vi "CLD 10 CSV file utility_exercise.vi"(8 "Error In":errorcluster, 10 "CLD 10 file Enum":T2, 11 "[Data In]":T1[](array[typedef])=[{"Step Time Target"=3, "Step 1"=TRUE, "Step 2"=FALSE, "Step 3"=FALSE}, {"Step Time Target"=4, "Step 1"=FALSE, "Step 2"=TRUE, "Step 3"=FALSE}, {"Step Time Target"=5, "Step 1"=FALSE, "Step 2"=FALSE, "Step 3"=TRUE}]) -> (0 "Error Out":errorcluster, 3 "[Data Out]":T1[](array[typedef]))   [LabVIEW 2025]
uses:
  CLD 10 CSV file data structure.ctl
  CLD 10 CSV file enum.ctl
  <vilib>/Utility/file.llb/Read Delimited Spreadsheet (string).vi
  <vilib>/Utility/file.llb/Write Delimited Spreadsheet (string).vi
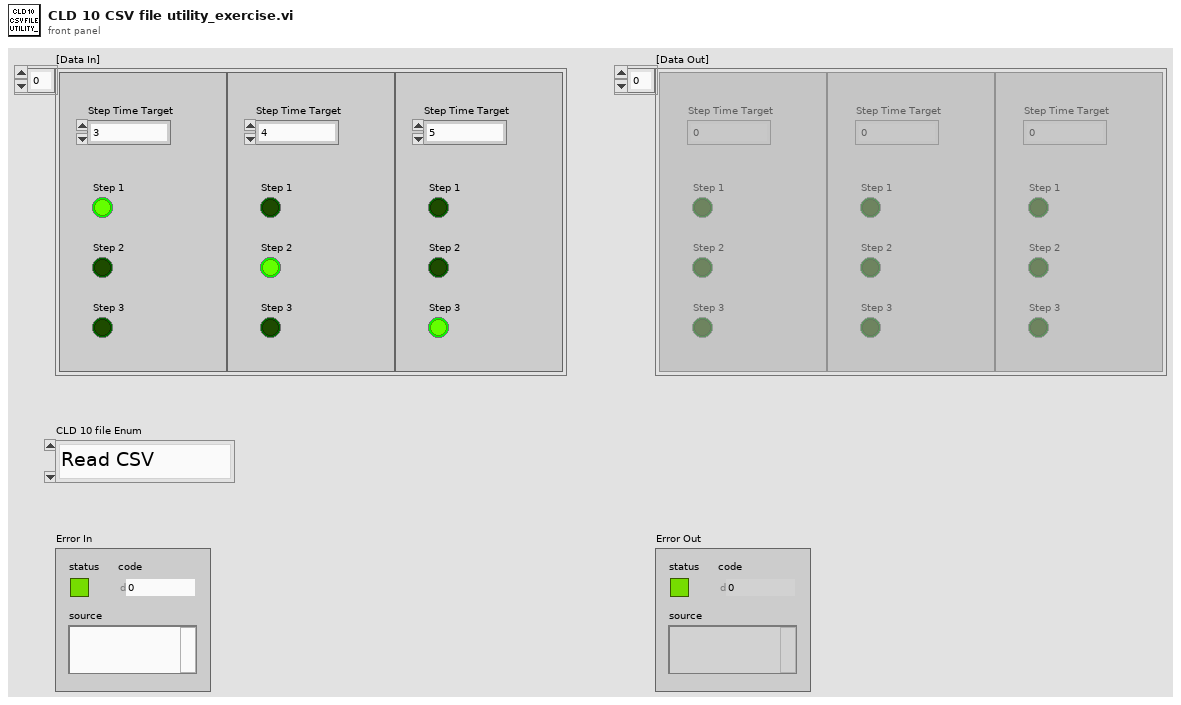
[diagram p1: front panel]
types:
  T1 = typedef "CLD 10 CSV file data structure.ctl" = cluster{"Step Time Target":i32, "Step 1":bool, "Step 2":bool, "Step 3":bool}
  T2 = typedef "CLD 10 CSV file enum.ctl" = enum16{"Read CSV", "Write CSV"}
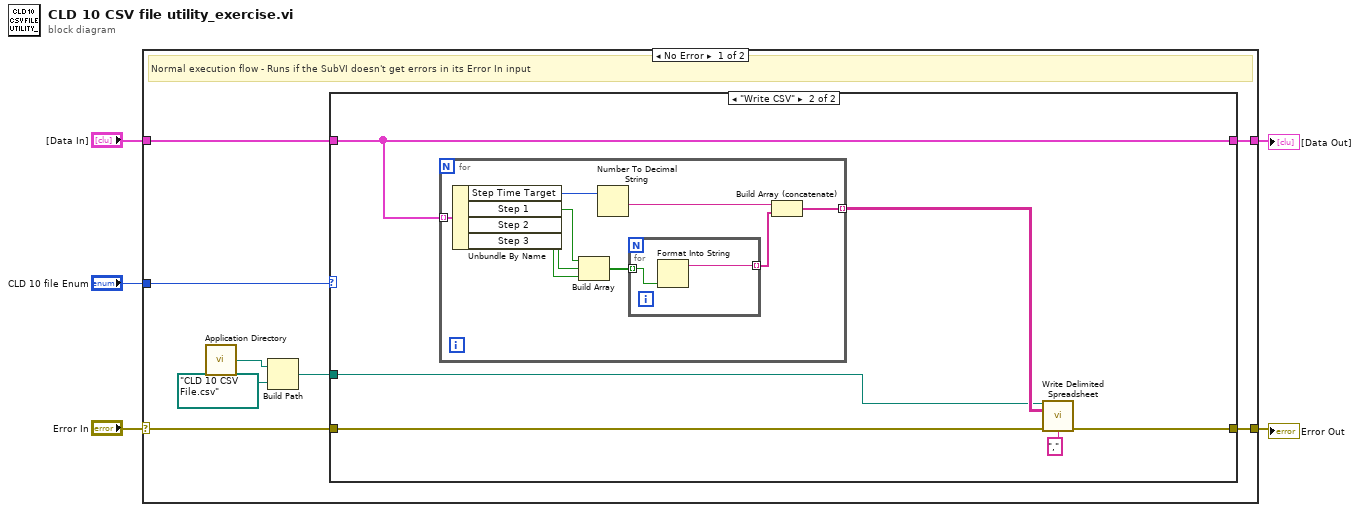
[diagram p0: block diagram]
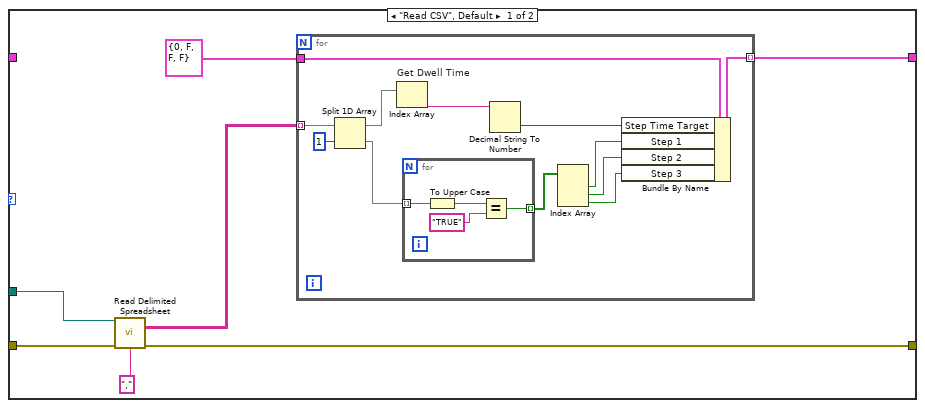
[diagram p2: hidden frame]
diagram:
  n1 = case shown="No Error" "Error In" {
    selector: "Error In" -> [w13 w55]
    tunnel: "[Data In]" -> [w12 w54]
    tunnel: [w11 w55] -> w3
    tunnel: [w10 w54] -> w2
    tunnel: "CLD 10 file Enum" -> [w9 _]
    frame No Error {
      # "Normal execution flow - Runs if the SubVI doesn't get errors in its Error In input"
      n2 = call <vilib>:"Application Directory.vi"() -> ("Application Directory"=w8:path)
      n3 = Build Path(base path=w8, name or relative path=path "CLD 10 CSV File.csv") -> (appended path=w6:path)
      n4 = case shown="\"Write CSV\"" w9 {
        tunnel: w13 -> [w20 w42]
        tunnel: w12 -> [_ w41]
        tunnel: [w19 w40] -> w11
        tunnel: [w15 w41] -> w10
        tunnel: w6 -> [w18 w38]
        frame "Read CSV", Default {
          n5 = call-poly <vilib>:"Read Delimited Spreadsheet.vi"("file path (dialog if empty)"=w18, "error in (no error)"=w20, "delimiter (\\t)"="," ("delimiter (\\t)")) -> ("all rows"=w17:string[][], "error out"=w19:errorcluster)  [unwired: 7 in, 4 out]
          n6 = for {
            tunnel: w17 -> [w32] mode=indexing
            tunnel: T1 {"Step Time Target"=0, "Step 1"=FALSE, "Step 2"=FALSE, "Step 3"=FALSE} ("CSV File Data Structure") -> [w30]
            tunnel: [w29] -> w15 mode=indexing
            n7 = Split 1D Array(array=w32, index=1) -> (first subarray=w31:string[], second subarray=w26:string[])
            n8 = Index Array "Get Dwell Time"(array=w31) -> (element=w27:string)  [unwired: 1 in]
            n9 = for {
              tunnel: w26 -> [w36] mode=indexing
              tunnel: [w33] -> w25 mode=indexing
              n10 = To Upper Case(1:w36) -> (0:w35:string)
              n11 = Equal?(x=w35, y="TRUE") -> (x = y?=w33:bool)
            }
            n12 = Decimal String To Number(string=w27) -> (number=w28:i32)  [unwired: 2 in, 1 out]
            n13 = Index Array(array=w25) -> (element #1=w24:bool, element #2=w23:bool, element #3=w22:bool)  [unwired: 3 in]
            n14 = Bundle By Name(cluster=w30, "Step Time Target"=w28, "Step 1"=w24, "Step 2"=w23, "Step 3"=w22) -> (w29:T1)
          }
        }
        frame "Write CSV" {
          n15 = for {
            tunnel: w41 -> [w51] mode=indexing
            tunnel: [w43] -> w39 mode=indexing
            n16 = Unbundle By Name(w51) -> ("Step Time Target"=w50:i32, "Step 1"=w49:bool, "Step 2"=w48:bool, "Step 3"=w47:bool)
            n17 = Build Array(w49, w48, w47) -> (w46:bool[])
            n18 = Number To Decimal String(number=w50) -> (decimal integer string=w44:string)  [unwired: 1 in]
            n19 = for {
              tunnel: w46 -> [w52] mode=indexing
              tunnel: [w53] -> w45 mode=indexing
              n20 = Format Into String "Format Into String"(w52) -> (resulting string=w53:string)  [unwired: 3 in, 1 out]
            }
            n21 = Build Array (concatenate)(w44, w45) -> (w43:string[])
          }
          n22 = call-poly <vilib>:"Write Delimited Spreadsheet.vi"("file path (dialog if empty)"=w38, "2D data"=w39, "error in (no error)"=w42, "delimiter (\\t)"="," ("delimiter (\\t)")) -> ("error out"=w40:errorcluster)  [unwired: 10 in, 1 out]
        }
      }
    }
    frame Error {
      # "Error execution flow - Determines how the SubVI responds if it gets errors in its Error In input"
    }
  }
  "[Data Out]" <- w2
  "Error Out" <- w3
